vi "Target Heading.vi"(10 "Target":dbl[](array[numeric]), 11 "Position":dbl[](array[numeric])) -> (3 "Heading (rad)":dbl format="%#_13g")   [LabVIEW 2016]
uses:
  <vilib>/Analysis/coordinate.llb/Angle Units.ctl
  <vilib>/Analysis/coordinate.llb/Angle Range (Degree).ctl
  <vilib>/Analysis/coordinate.llb/Wrap Angle (scalar).vi
  <vilib>/Analysis/NI_AAL_Angle.lvlib
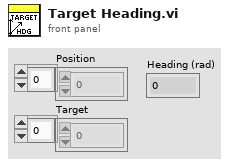
[diagram p1: front panel]
types:
  T1 = typedef "NI_AAL_Angle.lvlib/Angle Range (Degree).ctl" = u16
  T2 = typedef "NI_AAL_Angle.lvlib/Angle Units.ctl" = i32
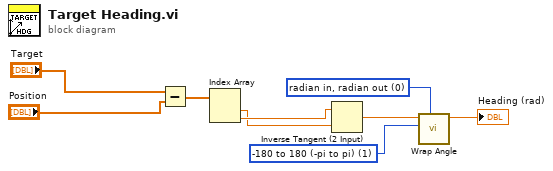
[diagram p0: block diagram]
diagram:
  w2 = T1 1 items=["none", "-180 to 180 (-pi to pi)", "0 to 360 (0 to 2pi)"] ("angle range")
  w3 = T2 0 items=["radian in, radian out", "radian in, degree out", "degree in, degree out", "degree in, radian out"] ("angle units")
  n1 = Subtract(x="Target", y="Position") -> (x-y=w7:dbl[])
  n2 = Index Array(array=w7) -> (element #1=w5:dbl, element #2=w6:dbl)  [unwired: 2 in]
  n3 = Inverse Tangent (2 Input)(1:w5, 2:w6) -> (0:w4:dbl)
  n4 = call-poly <vilib>:"Wrap Angle.vi"("angle units"=w3, "angle range"=w2, "angle in"=w4) -> ("angle out"=→"Heading (rad)":dbl)  [unwired: 7 in, 1 out]
